vi "Finalize.vi"(8 "error in":errorcluster, 11 "Plugin in":refnum<class "Analog Tachometer Process.lvclass">) -> (0 "error out":errorcluster, 3 "Plugin out":refnum<class "Analog Tachometer Process.lvclass">)   [LabVIEW 2025, in "Analog Tachometer Process.lvlib" / "Analog Tachometer Process.lvclass"]
uses:
  Analog Tachometer Process.lvclass
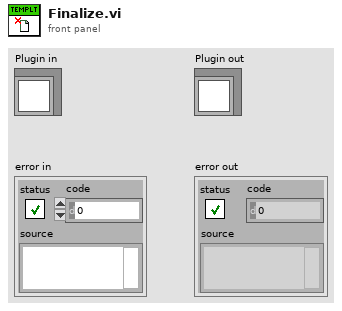
[diagram p1: front panel]
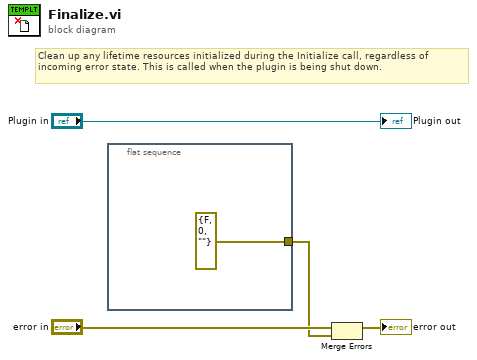
[diagram p0: block diagram]
diagram:
  # "Clean up any lifetime resources initialized during the Initialize call, regardless of incoming error state. This is called when the plugin is being shut down."
  n1 = flat-sequence {
    tunnel: [errorcluster {"status"=FALSE, "code"=0, "source"=""} ("error in")] -> w1
    frame #0 {
    }
  }
  n2 = Merge Errors("error in", w1) -> (→"error out":errorcluster)
  "Plugin out" <- "Plugin in"
